vi "SetBitfiledValue(DBL).vi"(8 "error in (no error)":errorcluster, 9 "bitfield value":dbl, 10 "bitfield caps":T1={"offset"=0, "size"=0, "signed?"=TRUE}, 11 "original value":u64 format="%.0x") -> (0 "error out":errorcluster, 3 "update value":u64 format="%.0x")   [LabVIEW 2017, in "Bitfield.lvlib"]
uses:
  Bitfield.lvlib
  BitfieldCaps.ctl
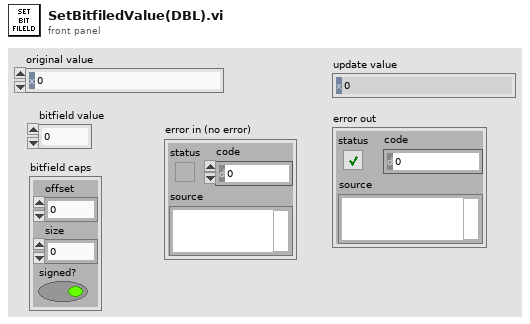
[diagram p1: front panel]
types:
  T1 = typedef "Bitfield.lvlib/BitfieldCaps.ctl" = cluster{"offset":i32, "size":i32, "signed?":bool}
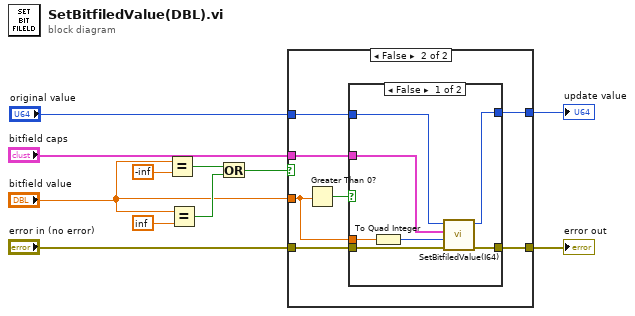
[diagram p0: block diagram]
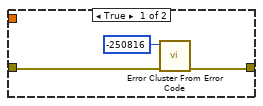
[diagram p2: hidden frame]
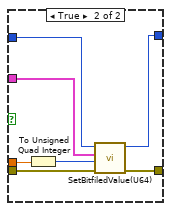
[diagram p3: hidden frame]
diagram:
  n1 = Equal?(x="bitfield value", y=-inf) -> (x = y?=w4:bool)
  n2 = Equal?(x="bitfield value", y=inf) -> (x = y?=w3:bool)
  n3 = Or(x=w4, y=w3) -> (x .or. y?=w2:bool)
  n4 = case shown="False" w2 {
    tunnel: "original value" -> [_ w21]
    tunnel: "bitfield caps" -> [_ w20]
    tunnel: "error in (no error)" -> [w13 w19]
    tunnel: [_ w18] -> w8
    tunnel: [w12 w17] -> w7
    tunnel: "bitfield value" -> [_ w15]
    frame True {
      n5 = call <vilib>:"Error Cluster From Error Code.vi"("error in (no error)"=w13, "error code (0)"=-250816) -> ("error out"=w12:errorcluster)  [unwired: 7 in]
    }
    frame False {
      n6 = Greater Than 0?(x=w15) -> (x > 0?=w16:bool)
      n7 = case shown="False" w16 {
        tunnel: w21 -> [w26 w35]
        tunnel: w20 -> [w25 w34]
        tunnel: w19 -> [w28 w33]
        tunnel: [w24 w32] -> w18
        tunnel: [w27 w31] -> w17
        tunnel: w15 -> [w23 w30]
        frame False {
          n8 = To Quad Integer(1:w23) -> (0:w22:i64)
          n9 = call "SetBitfiledValue(I64).vi"("error in (no error)"=w28, "bitfield value"=w22, "bitfield caps"=w25, "original value"=w26) -> ("error out"=w27:errorcluster, "update value"=w24:u64)  [unwired: 6 in]
        }
        frame True {
          n10 = To Unsigned Quad Integer(1:w30) -> (0:w29:u64)
          n11 = call "SetBitfiledValue(U64).vi"("error in (no error)"=w33, "bitfield value"=w29, "bitfield caps"=w34, "original value"=w35) -> ("error out"=w31:errorcluster, "update value"=w32:u64)  [unwired: 6 in]
        }
      }
    }
  }
  "update value" <- w8
  "error out" <- w7
